vi "Estimador del torque subVI.vi"(7 "Real":dbl, 8 "error in (no error)":errorcluster, 9 "Real 2":dbl, 10 "Real 3":dbl, 11 "appended path":path) -> (0 "error out":errorcluster, 3 "Numeric":dbl)   [LabVIEW 2019]
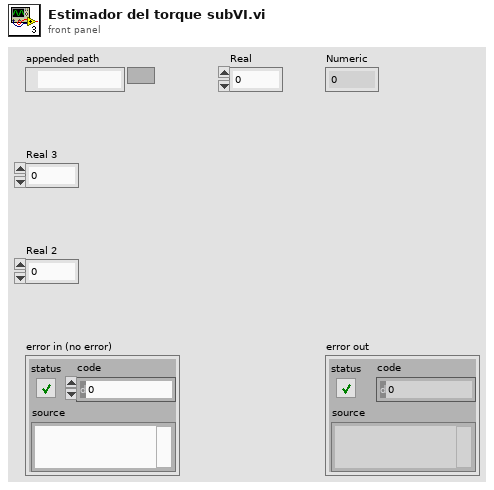
[diagram p1: front panel]
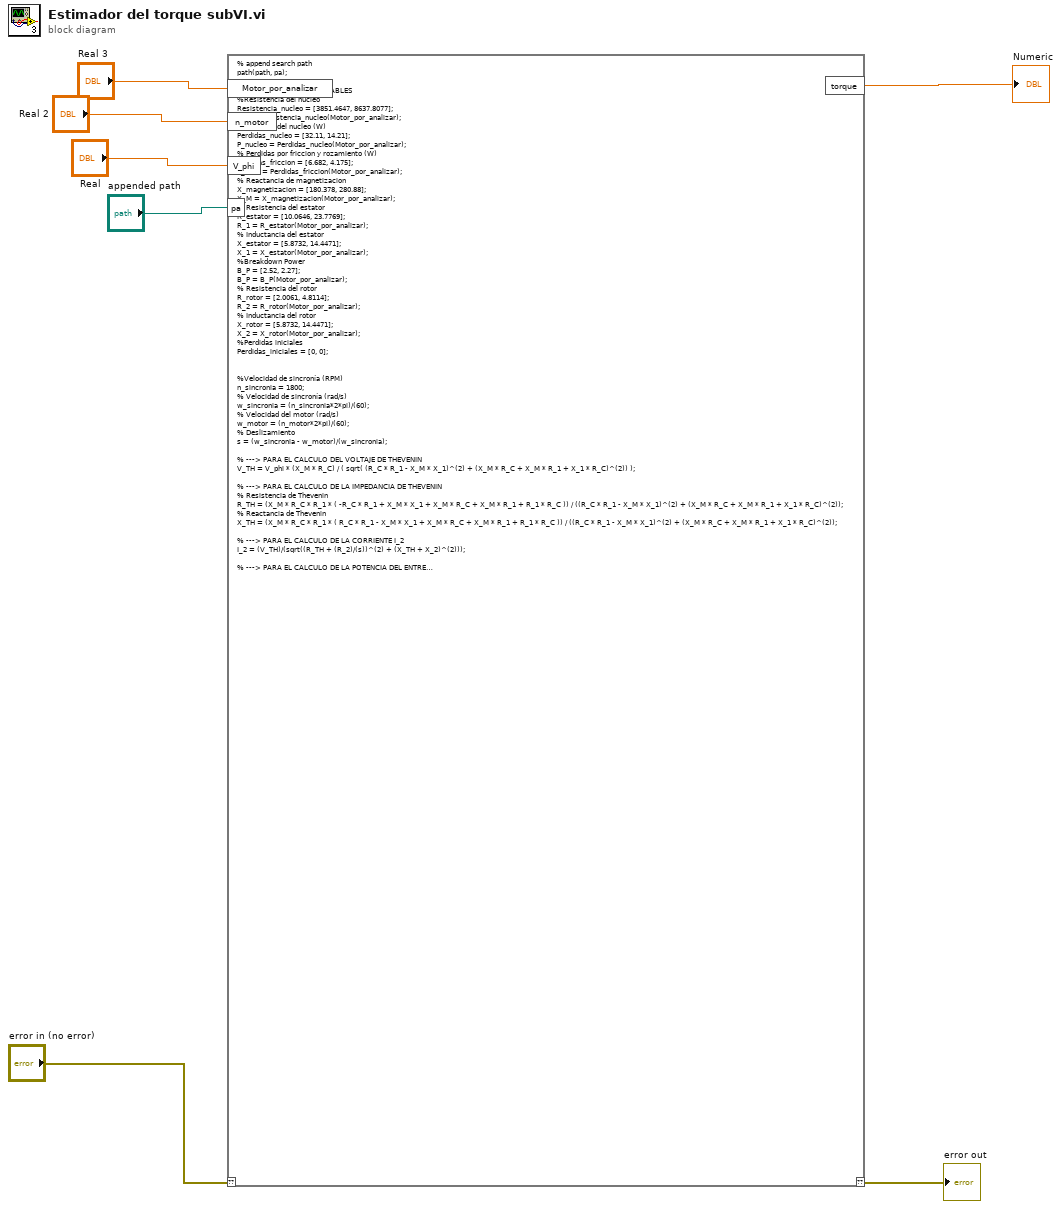
[diagram p0: block diagram]
diagram:
  n1 = script code="% append search path\npath(path, pa);\n\n% ---> SE DECLARAN VARIABLES\n%Resistencia del nucleo\nResistencia_nucleo = [3851.4647, 8637.8077];\nR_C = Resistencia_nucleo(Motor_por_analizar);\n% Perdidas del nucleo (W)\nPerdidas_nucleo = [32.11, 14.21];\nP_nucleo = Perdidas_nucleo(Motor_por_analizar);   \n% Perdidas por friccion y rozamiento (W)\nPerdidas_friccion = [6.682, 4.175];\nP_FyW = Perdidas_friccion(Motor_por_analizar);\n% Reactancia de magnetizacion\nX_magnetizacion = [180.378, 280.88];\nX_M = X_magnetizacion(Motor_por_analizar);\n% Resistencia del estator\nR_estator = [10.0646, 23.7769];\nR_1 = R_estator(Motor_por_analizar);\n% Inductancia del estator\nX_estator = [5.8732, 14.4471];\nX_1 = X_estator(Motor_por_analizar);\n%Breakdown Power\nB_P = [2.52, 2.27];\nB_P = B_P(Motor_por_analizar);\n% Resistencia del rotor\nR_rotor = [2.0061, 4.8114];\nR_2 = R_rotor(Motor_por_analizar);\n% Inductancia del rotor\nX_rotor = [5.8732, 14.4471];\nX_2 = X_rotor(Motor_por_analizar);\n%Perdidas iniciales\nPerdidas_iniciales = [0, 0];\n\n\n%Velocidad de sincronía (RPM)\nn_sincronia = 1800;\n% Velocidad de sincronía (rad/s)\nw_sincronia = (n_sincronia*2*pi)/(60);\n% Velocidad del motor (rad/s)\nw_motor = (n_motor*2*pi)/(60);\n% Deslizamiento\ns = (w_sincronia - w_motor)/(w_sincronia);\n\n% ---> PARA EL CALCULO DEL VOLTAJE DE THEVENIN\nV_TH = V_phi * (X_M * R_C) / ( sqrt( (R_C * R_1 - X_M * X_1)^(2) + (X_M * R_C + X_M * R_1 + X_1 * R_C)^(2)) );\n\n% ---> PARA EL CALCULO DE LA IMPEDANCIA DE THEVENIN\n% Resistencia de Thevenin\nR_TH = (X_M * R_C * R_1 * ( -R_C * R_1 + X_M * X_1 + X_M * R_C + X_M * R_1 + R_1 * R_C )) / ((R_C * R_1 - X_M * X_1)^(2) + (X_M * R_C + X_M * R_1 + X_1 * R_C)^(2));\n% Reactancia de Thevenin\nX_TH = (X_M * R_C * R_1 * ( R_C * R_1 - X_M * X_1 + X_M * R_C + X_M * R_1 + R_1 * R_C )) / ((R_C * R_1 - X_M * X_1)^(2) + (X_M * R_C + X_M * R_1 + X_1 * R_C)^(2));\n\n% ---> PARA EL CALCULO DE LA CORRIENTE I_2\nI_2 = (V_TH)/(sqrt((R_TH + (R_2)/(s))^(2) + (X_TH + X_2)^(2)));\n\n% ---> PARA EL CALCULO DE LA POTENCIA DEL ENTREHIERRO\nP_AG = 3/B_P * (I_2)^2 * (R_2)/(s);\n\n% ---> PARA EL CALCULO DEL TORQUE INDUCIDO\nT_ind = (P_AG)/(w_sincronia);\n\n% ---> PARA EL CALCULO DEL TORQUE EN LA CARGA\n% Perdidas rotacionales\nP_rot = P_FyW;\n% Perdidas de torque\nT_perdidas = ((P_rot)*(1 - s))/(w_motor);\n% Torque en la carga (N*m)\n\nif T_perdidas >= Perdidas_iniciales(Motor_por_analizar)\n    T_carga = T_ind - T_perdidas;\nelse \n    T_carga = T_ind - Perdidas_iniciales(Motor_por_analizar);\nend\n\nif n_motor == 1800\n    T_carga = 0;\nend\n\ntorque = T_carga;"("??"="error in (no error)", "Motor_por_analizar"="Real 3", "n_motor"="Real 2", "V_phi"="Real", "pa"="appended path") -> ("??"=→"error out":errorcluster, "torque"=→"Numeric":dbl)
